vi "GetAVICodecs.vi"(6 "error in (no error)":errorcluster, 7 "Refnum in":T1, 8 "Bit Depth":u32, 9 "Format":u32, 10 "Height":u32, 11 "Width":u32) -> (0 "error out":errorcluster, 3 "Codec Names":string[](array[string]))   [LabVIEW 2023]
uses:
  <vilib>/vision/Image Controls.llb/IMAQ Image.ctl
  <vilib>/vision/Avi.llb/IMAQ AVI2 Codec Path.ctl
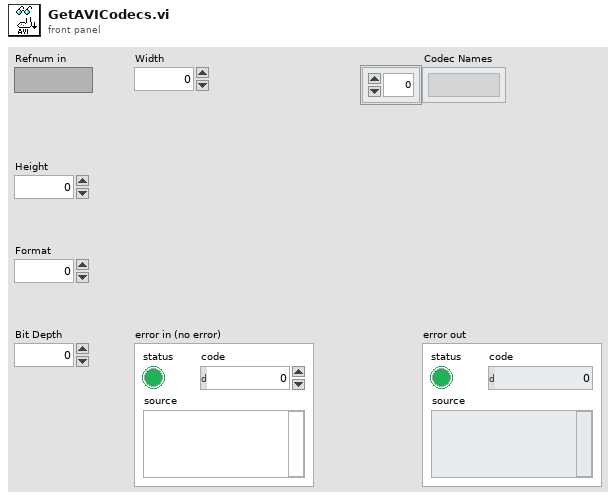
[diagram p1: front panel]
types:
  T1 = typedef "IMAQ Image.ctl" = refnum<image>
  T2 = typedef "IMAQ AVI2 Codec Path.ctl" = u32
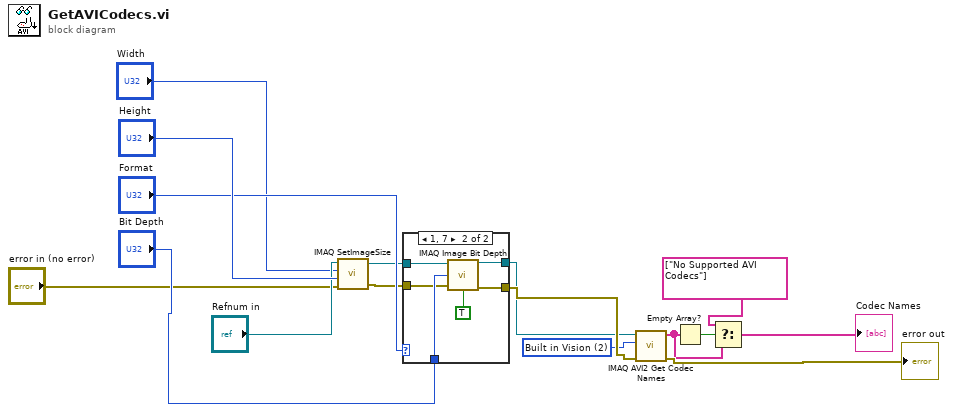
[diagram p0: block diagram]
diagram:
  w11 = T2 2 items=["Default", "System", "Built in Vision"] ("Codec Source")
  n1 = call "IMAQ SetImageSize"("error in (no error)"="error in (no error)", "Y Resolution"="Height", "X Resolution"="Width", "Image"="Refnum in") -> ("error out"=w4:errorcluster, "Image Out"=w3:T1)  [unwired: 1 in]
  n2 = case shown="1, 7" "Format" {
    tunnel: [w17 w24] -> w12
    tunnel: "Bit Depth" -> [_ w23]
    tunnel: w4 -> [w17 w22]
    tunnel: w3 -> [w18 w20]
    tunnel: [w18 w19] -> w10
    frame 0, Default {
    }
    frame 1, 7 {
      n3 = call "IMAQ Image Bit Depth"("Image"=w20, "Bit Depth (0)"=w23, "error in (no error)"=w22, "Get/Set Bit Depth? (Set)"=TRUE) -> ("Image Out"=w19:T1, "error out"=w24:errorcluster)  [unwired: 9 in, 1 out]
    }
  }
  n4 = call "IMAQ AVI2 Get Codec Names"("error in (no error)"=w12, "Codec Source"=w11, "Image"=w10) -> ("error out"=→"error out":errorcluster, "Codec Names"=w7:string[])  [unwired: 7 in]
  n5 = Empty Array?(array=w7) -> (empty?=w8:bool)
  n6 = Select(t=string[] ["No Supported AVI Codecs"], s=w8, f=w7) -> (s? t:f=→"Codec Names":string[])
